vi "Create Test Suite (AllAsserts).vi.vi"(5 "Interactive (T)":bool=TRUE, 7 "Verbose (F)":bool, 8 "error in (no error)":errorcluster, 9 "Test Report":refnum<class "Test Report.lvclass">, 11 "Test Runner.AllAsserts out":refnum<class "Test Runner.AllAsserts.lvclass">) -> (0 "error out":errorcluster, 3 "Test Runner.AllAsserts in":refnum<class "Test Runner.AllAsserts.lvclass">)   [LabVIEW 2013, in "Test Runner.AllAsserts.lvclass"]
uses:
  Test Runner.AllAsserts.lvclass
  classes/Test Report/Test Report.lvclass
  classes/Test Runner/Test Runner.lvclass/Test Runner.ctl
  classes/Test Runner/Test Runner.lvclass
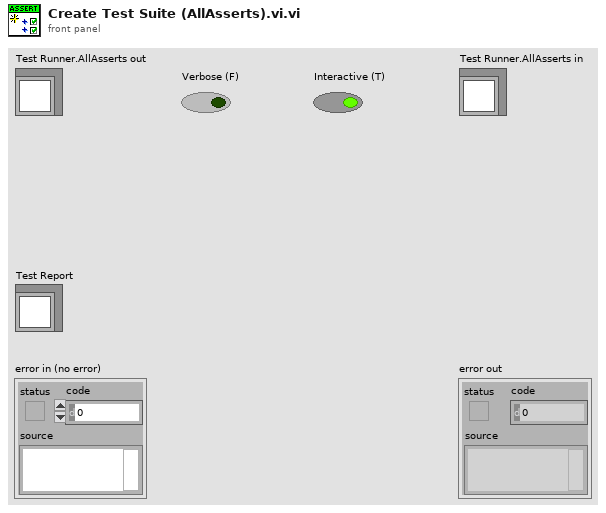
[diagram p1: front panel]
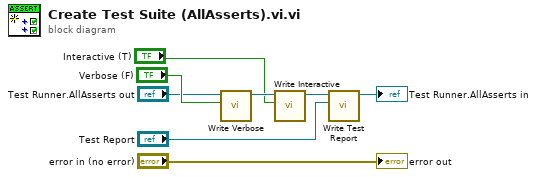
[diagram p0: block diagram]
diagram:
  n1 = call "Write Verbose.vi"("Verbose"="Verbose (F)", "Test Runner in"="Test Runner.AllAsserts out") -> ("Test Runner out"=w6:refnum<class "Test Runner.AllAsserts.lvclass">)  [unwired: 9 in]
  n2 = call "Write Interactive.vi"("Interactive"="Interactive (T)", "Test Runner in"=w6) -> ("Test Runner out"=w3:refnum<class "Test Runner.AllAsserts.lvclass">)  [unwired: 9 in]
  n3 = call "Write Test Report.vi"("Test Report"="Test Report", "Test Runner in"=w3) -> ("Test Runner out"=→"Test Runner.AllAsserts in":refnum<class "Test Runner.AllAsserts.lvclass">)  [unwired: 9 in]
  "error out" <- "error in (no error)"
